vi "GrabImageDisplay.vi"(2 "error in (no error)":errorcluster, 3 "Image Src":T1, 4 "IBaseData":refnum<k24>) -> (0 "error out":errorcluster, 1 "Image out":T1)   [LabVIEW 2013, in "GxLVlib.lvlib"]
uses:
  GxLVlib.lvlib
  F:/GxILibrary/Labview/trunk/private/dev/src/C#/x86/GxLVLib/dll/GxIAPINET.dll
  private/dev/src/C#/x86/GxLVLib/dll/GxIAPINET.dll
  <vilib>/vision/Image Controls.llb/IMAQ Image.ctl
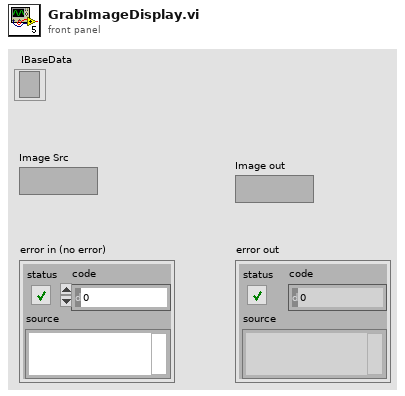
[diagram p1: front panel]
types:
  T1 = typedef "IMAQ Image.ctl" = refnum<image>
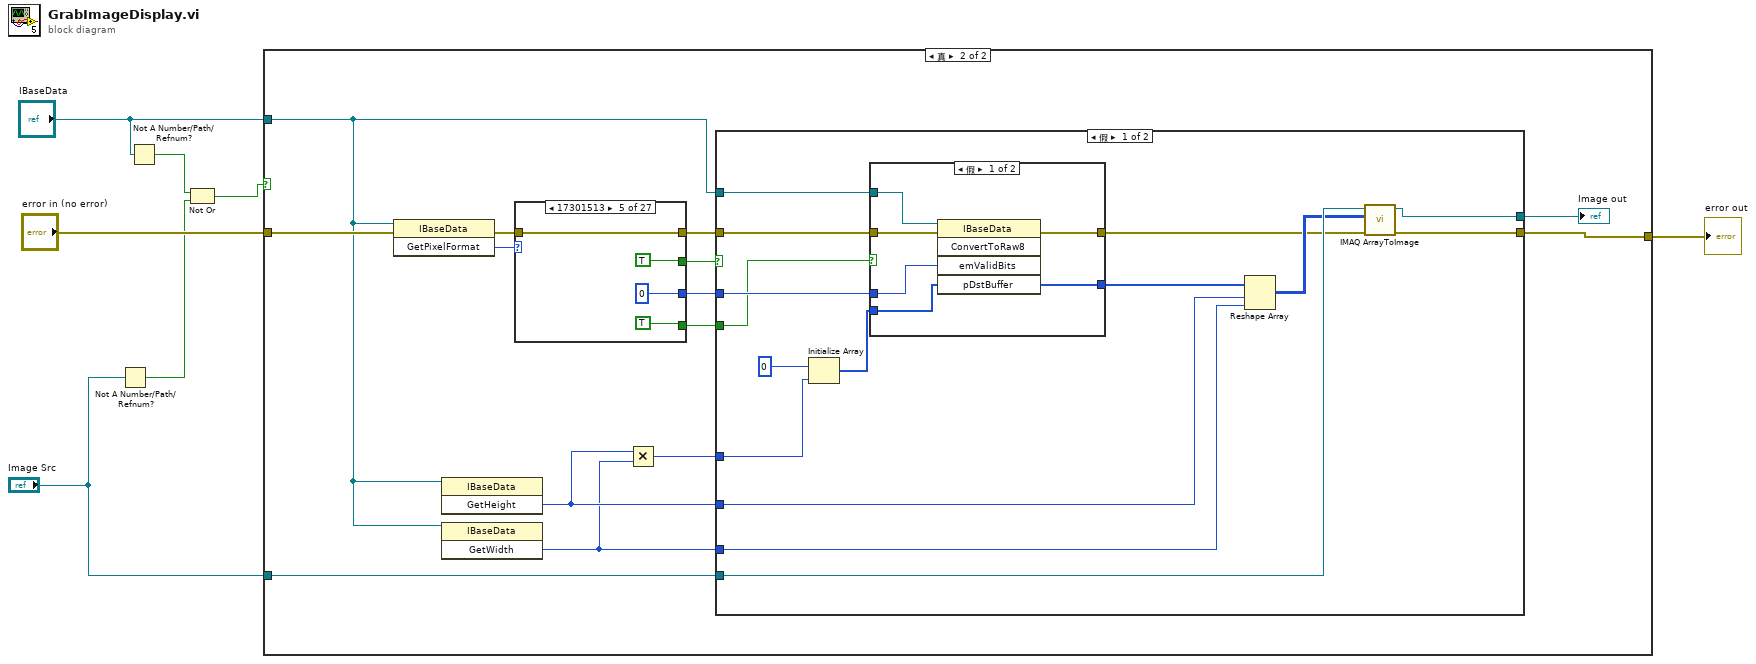
[diagram p0: block diagram]
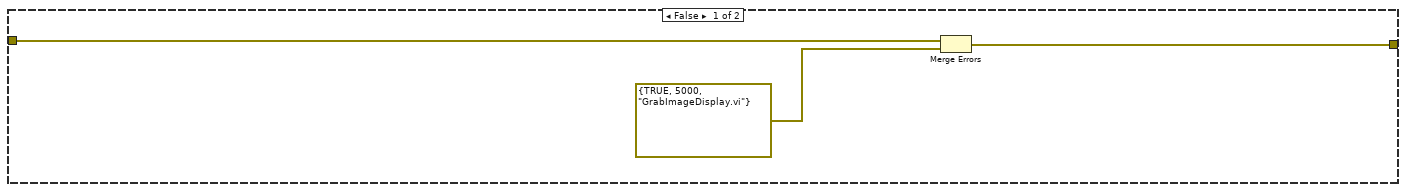
[diagram p2: hidden frame]
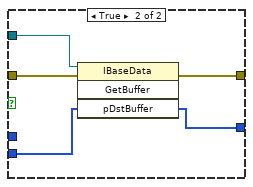
[diagram p3: hidden frame]
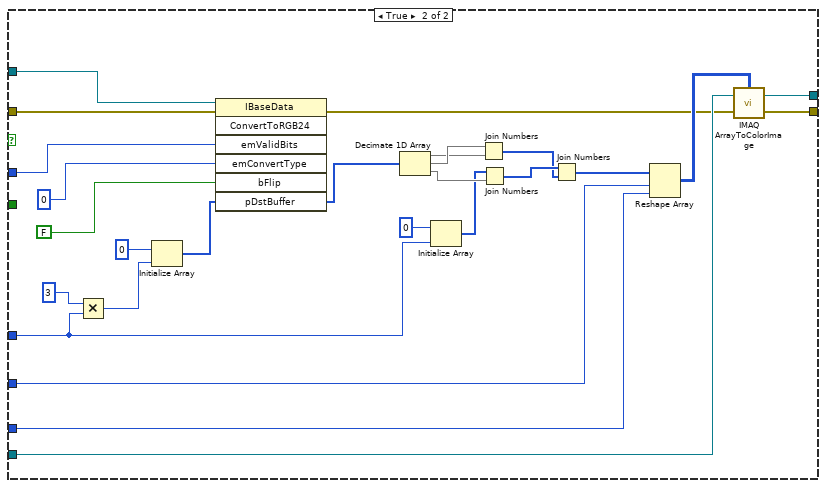
[diagram p4: hidden frame]
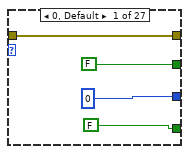
[diagram p5: hidden frame]
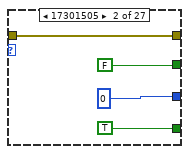
[diagram p6: hidden frame]
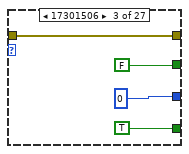
[diagram p7: hidden frame]
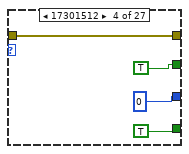
[diagram p8: hidden frame]
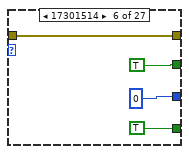
[diagram p9: hidden frame]
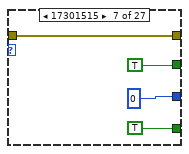
[diagram p10: hidden frame]
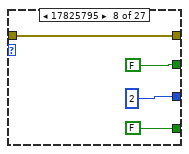
[diagram p11: hidden frame]
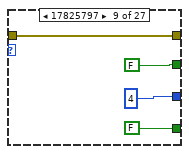
[diagram p12: hidden frame]
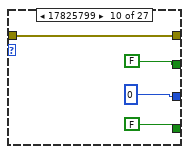
[diagram p13: hidden frame]
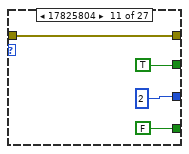
[diagram p14: hidden frame]
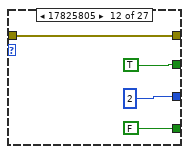
[diagram p15: hidden frame]
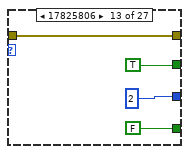
[diagram p16: hidden frame]
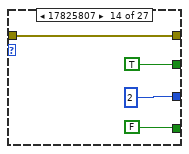
[diagram p17: hidden frame]
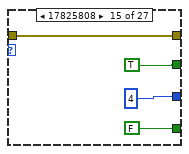
[diagram p18: hidden frame]
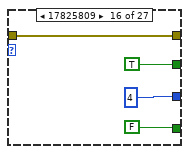
[diagram p19: hidden frame]
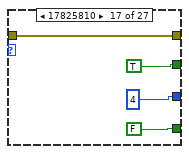
[diagram p20: hidden frame]
diagram:
  n1 = Not A Number/Path/Refnum?(number/path/refnum="Image Src") -> (NaN/Path/Refnum?=w3:bool)
  n2 = Not A Number/Path/Refnum?(number/path/refnum="IBaseData") -> (NaN/Path/Refnum?=w2:bool)
  n3 = Not Or(1:w3, 2:w2) -> (0:w1:bool)
  n4 = case shown="真" w1 {
    tunnel: "IBaseData" -> [_ w14]
    tunnel: "error in (no error)" -> [w10 w22]
    tunnel: [w8 w16] -> w5
    tunnel: "Image Src" -> [_ w17]
    frame False {
      n5 = Merge Errors(w10, errorcluster {TRUE, 5000, "GrabImageDisplay.vi"}) -> (w8:errorcluster)
    }
    frame True {
      n6 = invoke class="IBaseData" method="GetPixelFormat"(reference=w14, error in=w22) -> (error out=w19:errorcluster, "GetPixelFormat"=w21:u32)  [unwired: 1 in, 1 out]
      n7 = invoke class="IBaseData" method="GetHeight"(reference=w14) -> ("GetHeight"=w12:u64)  [unwired: 2 in, 2 out]
      n8 = invoke class="IBaseData" method="GetWidth"(reference=w14) -> ("GetWidth"=w11:u64)  [unwired: 2 in, 2 out]
      n9 = case shown="17301513" w21 {
        tunnel: [0 0 0 0 0 0 0 2 4 0 2 2 2 2 4 4 4 4 0 0 0 0 0 0 2 4 0] -> w23
        tunnel: [FALSE FALSE FALSE TRUE TRUE TRUE TRUE FALSE FALSE FALSE TRUE TRUE TRUE TRUE TRUE TRUE TRUE TRUE FALSE TRUE TRUE TRUE TRUE TRUE TRUE TRUE TRUE] -> w24
        tunnel: [FALSE TRUE TRUE TRUE TRUE TRUE TRUE FALSE FALSE FALSE FALSE FALSE FALSE FALSE FALSE FALSE FALSE FALSE FALSE FALSE FALSE FALSE FALSE FALSE FALSE FALSE FALSE] -> w20
        tunnel: w19 -> [w77 w81 w88 w92 w96 w100 w104 w108 w112 w116 w120 w124 w128 w132 w136 w140 w144 w148 w152 w156 w160 w164 w168 w172 w176 w180 w184]
        tunnel: [w77 w81 w88 w92 w96 w100 w104 w108 w112 w116 w120 w124 w128 w132 w136 w140 w144 w148 w152 w156 w160 w164 w168 w172 w176 w180 w184] -> w18
        frame 0, Default {
        }
        frame 17301505 {
        }
        frame 17301506 {
        }
        frame 17301512 {
        }
        frame 17301513 {
        }
        frame 17301514 {
        }
        frame 17301515 {
        }
        frame 17825795 {
        }
        frame 17825797 {
        }
        frame 17825799 {
        }
        frame 17825804 {
        }
        frame 17825805 {
        }
        frame 17825806 {
        }
        frame 17825807 {
        }
        frame 17825808 {
        }
        frame 17825809 {
        }
        frame 17825810 {
        }
        frame 17825811 {
        }
        frame 17825829 {
        }
        frame 17825838 {
        }
        frame 17825839 {
        }
        frame 17825840 {
        }
        frame 17825841 {
        }
        frame 35127329 {
        }
        frame 36700194 {
        }
        frame 36700195 {
        }
        frame 36700196 {
        }
      }
      n10 = Multiply(x=w12, y=w11) -> (x*y=w13:u64)
      n11 = case shown="假" w24 {
        tunnel: w23 -> [w39 w76]
        tunnel: w13 -> [w37 w60]
        tunnel: w20 -> [w35 _]
        tunnel: w14 -> [w36 w71]
        tunnel: w18 -> [w34 w70]
        tunnel: w17 -> [w33 w68]
        tunnel: [w31 w66] -> w16
        tunnel: [w28 w67] -> w15
        tunnel: w12 -> [w30 w65]
        tunnel: w11 -> [w29 w64]
        frame False {
          n12 = Initialize Array(u8 0, w37) -> (w27:u8[])
          n13 = case shown="假" w35 {
            tunnel: w39 -> [w45 _]
            tunnel: w36 -> [w44 w50]
            tunnel: w34 -> [w43 w49]
            tunnel: [w42 w48] -> w25
            tunnel: w27 -> [w41 w47]
            tunnel: [w40 w46] -> w26
            frame False {
              n14 = invoke class="IBaseData" method="ConvertToRaw8"(reference=w44, error in=w43, "emValidBits"=w45, "pDstBuffer"=w41) -> (error out=w42:errorcluster, "pDstBuffer"=w40:u8[])  [unwired: 1 in, 3 out]
            }
            frame True {
              n15 = invoke class="IBaseData" method="GetBuffer"(reference=w50, error in=w49, "pDstBuffer"=w47) -> (error out=w48:errorcluster, "pDstBuffer"=w46:u8[])  [unwired: 1 in, 2 out]
            }
          }
          n16 = Reshape Array(w26, w30, w29) -> (w32:u8[][])
          n17 = call "IMAQ ArrayToImage"("error in (no error)"=w25, "Image Pixels (U8)"=w32, "Image"=w33) -> ("error out"=w31:errorcluster, "Image Out"=w28:T1)  [unwired: 7 in]
        }
        frame True {
          n18 = Multiply(x=3, y=w60) -> (x*y=w69:u64)
          n19 = Initialize Array(u8 0, w69) -> (w53:u8[])
          n20 = invoke class="IBaseData" method="ConvertToRGB24"(reference=w71, error in=w70, "emValidBits"=w76, "emConvertType"=0, "bFlip"=FALSE, "pDstBuffer"=w53) -> (error out=w51:errorcluster, "pDstBuffer"=w52:u8[])  [unwired: 1 in, 5 out]
          n21 = Decimate 1D Array(w52) -> (w58:u8[], w59:u8[], w57:u8[])
          n22 = Initialize Array(u8 0, w60) -> (w56:u8[])
          n23 = Join Numbers(hi=w59, lo=w58) -> ((hi.lo)=w54:u16[])
          n24 = Join Numbers(hi=w56, lo=w57) -> ((hi.lo)=w55:u16[])
          n25 = Join Numbers(hi=w55, lo=w54) -> ((hi.lo)=w62:u32[])
          n26 = Reshape Array(w62, w65, w64) -> (w63:u32[][])
          n27 = call "IMAQ ArrayToColorImage"("Image Pixels (U32)"=w63, "Image"=w68, "error in (no error)"=w51) -> ("Image Out"=w67:T1, "error out"=w66:errorcluster)  [unwired: 2 in]
        }
      }
      "Image out" <- w15
    }
  }
  "error out" <- w5
